vi "pump Status.vi"(0 "pumpIndex":u32, 1 "channel":u32, 2 "errorCode":i32, 3 "pumpState":i32, 4 "pumpRate":sgl, 5 "pressure":sgl, 6 "lastOverPressure":sgl, 7 "error in (no error)":errorcluster) -> (20 "function return":i32, 22 "errorCode out":i32, 23 "pumpState out":i32, 24 "pumpRate out":sgl, 25 "pressure out":sgl, 26 "lastOverPressure out":sgl, 27 "error out":errorcluster)   [LabVIEW 2018]
doc: "extern ASIAPUMP_INTERFACE_API BOOL pumpStatus(\n unsigned int pumpIndex ,\n unsigned int channel ,\n int * errorCode ,\n int * pumpState ,\n float * pumpRate ,\n float * pressure ,\n float * lastOverPressure \n );"
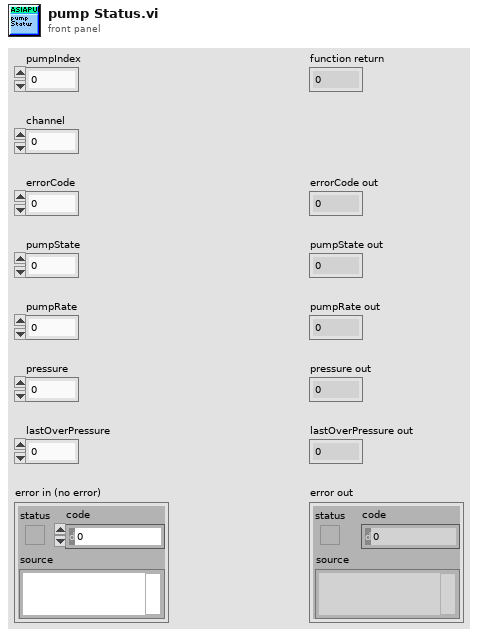
[diagram p1: front panel]
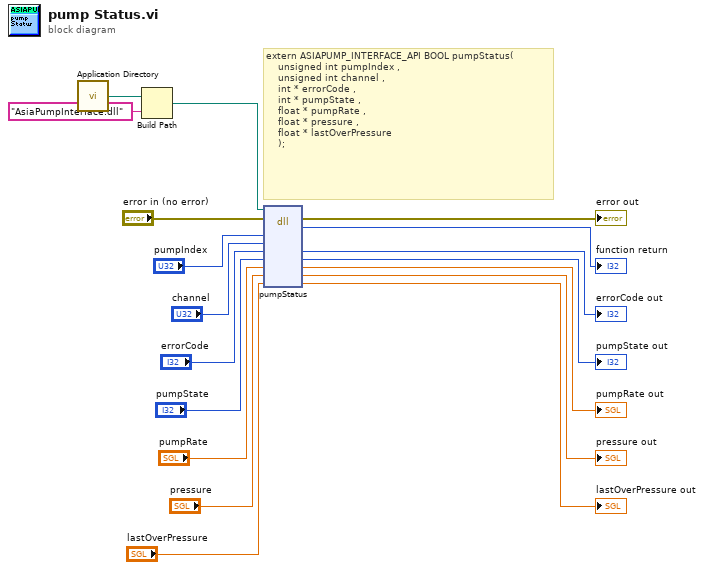
[diagram p0: block diagram]
diagram:
  # "extern ASIAPUMP_INTERFACE_API BOOL pumpStatus(\n    unsigned int pumpIndex ,\n    unsigned int channel ,\n    int * errorCode ,\n    int * pumpState ,\n    float * pumpRate ,\n    float * pressure ,\n    float * lastOverPressure \n    );"
  n1 = call <vilib>:"Application Directory.vi"() -> ("Application Directory"=w3:path)
  n2 = Build Path(base path=w3, name or relative path="AsiaPumpInterface.dll") -> (appended path=w1:path)
  n3 = dll-call lib="C:/Program Files (x86)/National Instruments/LabVIEW 2018/user.lib/AsiaPumpInterface/AsiaPumpInterface.*" fn="pumpStatus"(path in=w1, error in="error in (no error)", "pumpIndex"="pumpIndex", "channel"="channel", "errorCode"="errorCode", "pumpState"="pumpState", "pumpRate"="pumpRate", "pressure"="pressure", "lastOverPressure"="lastOverPressure") -> (error out=→"error out":errorcluster, "return type"=→"function return":i32, "errorCode"=→"errorCode out":i32, "pumpState"=→"pumpState out":i32, "pumpRate"=→"pumpRate out":sgl, "pressure"=→"pressure out":sgl, "lastOverPressure"=→"lastOverPressure out":sgl)  [unwired: 3 in, 1 out]
